vi "CAN_tester.vi"() -> ()   [LabVIEW 2017]
uses:
  <vilib>/nican/nican.llb/CanFrameTimed.ctl
panel:
  out "Frame to write":T1[](array[typedef]) {"Data" format="%.0x"; "ArbitrationId" format="%.0x"; "Timestamp" format="%<%I:%M:%S%3u %p\n%m/%d/%Y>T"}
  in  "Active":bool
  in  "Steering Control":T2={"Rot. sw 4"=1, "Rot. sw 5"=1, "Rot. sw 3"=1, "Rot. sw 1"=1, "Rot. sw 2"=1, "Button 3"=FALSE, "Button 1"=FALSE, "Button 2"=FALSE, "Button 4"=FALSE} {"Rot. sw 2" min=1 max=12 scale=1.0..12.0; "Rot. sw 1" min=1 max=12 scale=1.0..12.0; "Rot. sw 3" min=1 max=12 scale=1.0..12.0; "Rot. sw 5" min=1 max=12 scale=1.0..12.0; "Rot. sw 4" min=1 max=12 scale=1.0..12.0}
  in  "Brake Checked":T3 {"Brake Pressure Front" scale=0.0..100.0; "Brake Pressure Rear" scale=0.0..100.0}
  in  "Active":bool
  in  "AMK Setpoint FL":T4 {"AMK_Targetvelocity" scale=0.0..21500.0; "AMK_TorqueLimitPositive" scale=0.0..2140.0; "AMK_TorqueLimitNegative" scale=0.0..-2140.0}
  in  "Active":bool
  in  "AMK Setpoint RL":T4 {"AMK_Targetvelocity" scale=0.0..21500.0; "AMK_TorqueLimitPositive" scale=0.0..2140.0; "AMK_TorqueLimitNegative" scale=0.0..-2140.0}
  in  "Active":bool
  in  "AMK Setpoint FR":T4 {"AMK_Targetvelocity" scale=0.0..21500.0; "AMK_TorqueLimitPositive" scale=0.0..2140.0; "AMK_TorqueLimitNegative" scale=0.0..-2140.0}
  in  "Active":bool
  in  "AMK Setpoint FL":T4 {"AMK_Targetvelocity" scale=0.0..21500.0; "AMK_TorqueLimitPositive" scale=0.0..2140.0; "AMK_TorqueLimitNegative" scale=0.0..-2140.0}
  in  "Active":bool
  in  "Active":bool
  in  "ThrottleSteering":T5 {"APPS2" scale=0.0..100.0; "APPS1" scale=0.0..100.0; "Steering Angle 2" scale=90.0..-90.0; "Steering Angle 1" scale=90.0..-90.0}
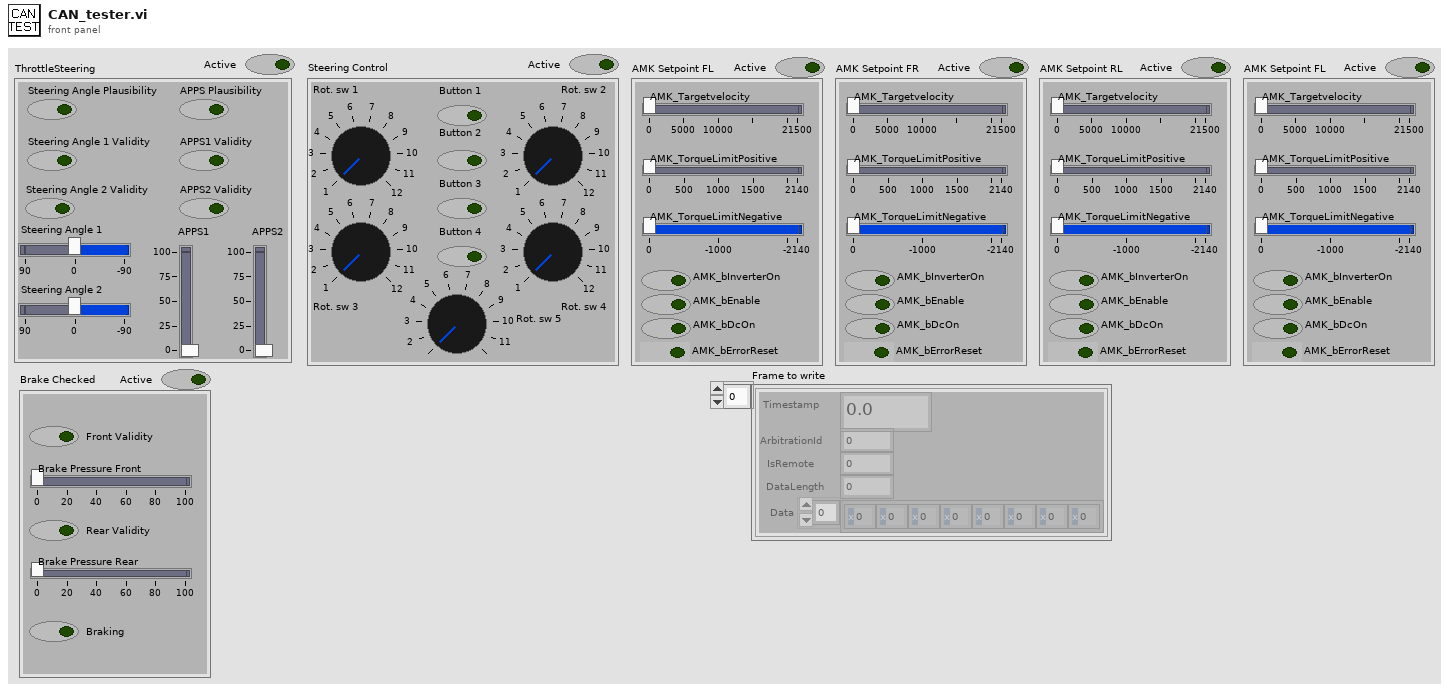
[diagram p1: front panel]
types:
  T1 = typedef "CanFrameTimed.ctl" = cluster{"Timestamp":dbl, "ArbitrationId":u32, "IsRemote":u8, "DataLength":u8, "Data":u8[]}
  T2 = cluster{"Rot. sw 4":u16, "Rot. sw 5":u16, "Rot. sw 3":u16, "Rot. sw 1":u16, "Rot. sw 2":u16, "Button 3":bool, "Button 1":bool, "Button 2":bool, "Button 4":bool}
  T3 = cluster{"Rear Validity":bool, "Front Validity":bool, "Brake Pressure Rear":dbl, "Brake Pressure Front":dbl, "Braking":bool}
  T4 = cluster{"AMK_bErrorReset":bool, "AMK_bDcOn":bool, "AMK_bEnable ":bool, "AMK_bInverterOn":bool, "AMK_TorqueLimitNegative":dbl, "AMK_TorqueLimitPositive":dbl, "AMK_Targetvelocity":dbl}
  T5 = cluster{"APPS Plausibility":bool, "Steering Angle 1":dbl, "Steering Angle 2":dbl, "APPS1":dbl, "APPS2":dbl, "APPS1 Validity":bool, "APPS2 Validity":bool, "Steering Angle Plausibility":bool, "Steering Angle 1 Validity":bool, "Steering Angle 2 Validity":bool}
  T6 = typedef "xobjhandle.ctl" = u32
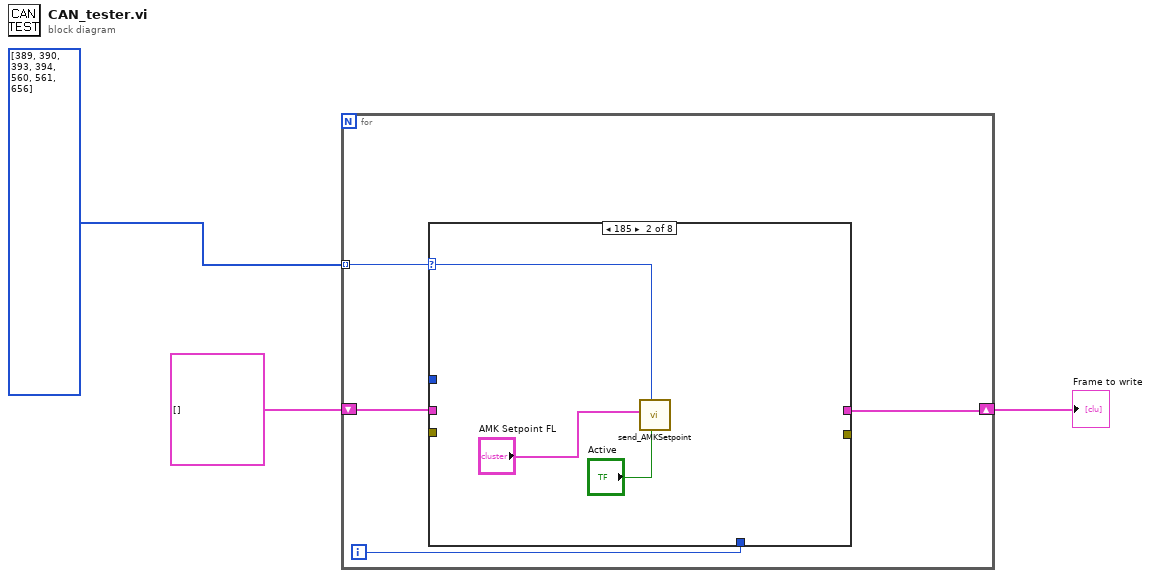
[diagram p0: block diagram]
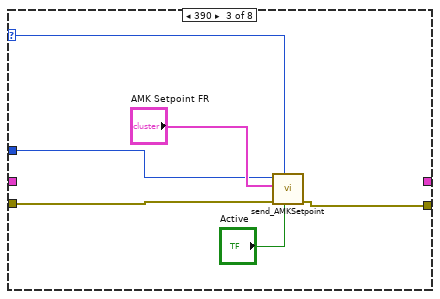
[diagram p3: hidden frame]
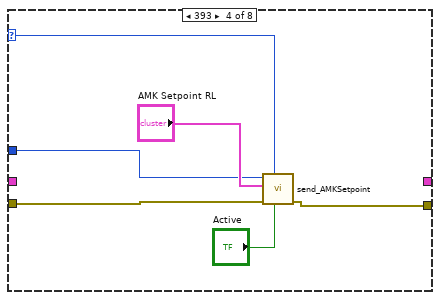
[diagram p4: hidden frame]
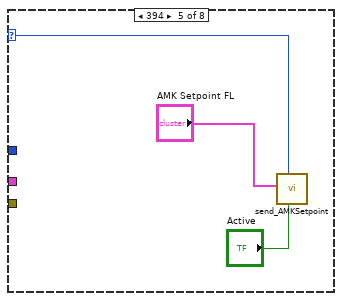
[diagram p5: hidden frame]
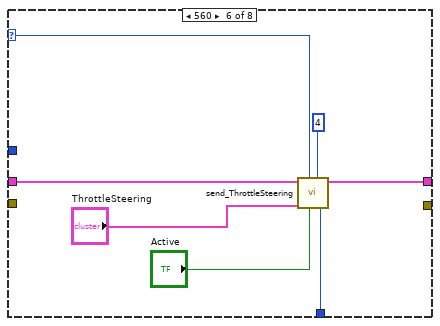
[diagram p6: hidden frame]
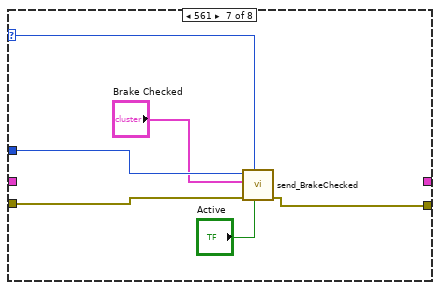
[diagram p7: hidden frame]
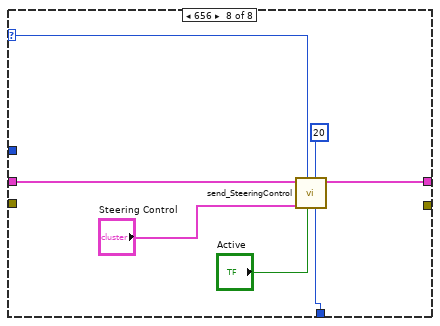
[diagram p8: hidden frame]
diagram:
  n1 = for {
    tunnel: u32[] [389, 390, 393, 394, 560, 561, 656] -> [w7] mode=indexing
    shift-right: [w5] -> w1
    shift-left: T1[] [] ("CAN frame") -> [w6]
    i -> [w4]
    n2 = case shown="185" w7 {
      selector: w7 -> [_ w9 w12 w19 w26 w34 w36 w49]
      tunnel: _ -> [_ _ w16 w22 _ _ w40 _]
      tunnel: [_ _ w13 w20 _ _ w41 _] -> _
      tunnel: _ -> [_ _ w15 w21 _ _ w39 _]
      tunnel: [w8 _ _ _ _ w33 _ w43] -> w5
      tunnel: w6 -> [w8 _ _ _ _ w31 _ w45]
      tunnel: w4 -> [_ _ _ _ _ w29 _ w47]
      frame 0, Default {
      }
      frame 389 {
        n3 = call "send_AMKSetpoint.vi"("Active"="Active", "ID"=w9, "Message"="AMK Setpoint FL") -> ()  [unwired: 7 in, 2 out]
      }
      frame 390 {
        n4 = call "send_AMKSetpoint.vi"("Active"="Active", "ID"=w12, "Error in"=w15, "Message"="AMK Setpoint FR", "ObjHandle in"=w16) -> ("Error out"=w13:errorcluster, "ObjHandle out"=w14:T6)  [unwired: 5 in]
      }
      frame 393 {
        n5 = call "send_AMKSetpoint.vi"("Active"="Active", "ID"=w19, "Error in"=w21, "Message"="AMK Setpoint RL", "ObjHandle in"=w22) -> ("Error out"=w20:errorcluster, "ObjHandle out"=w23:T6)  [unwired: 5 in]
      }
      frame 394 {
        n6 = call "send_AMKSetpoint.vi"("Active"="Active", "ID"=w26, "Message"="AMK Setpoint FL") -> ()  [unwired: 7 in, 2 out]
      }
      frame 560 {
        n7 = call "send_ThrottleSteering.vi"("Counter"=w29, "200/freq"=4, "Active"="Active", "CAN ID"=w34, "Message"="ThrottleSteering", "CAN frame"=w31) -> ("CAN frame out"=w33:T1[])  [unwired: 5 in]
      }
      frame 561 {
        n8 = call "send_BrakeChecked.vi"("Active"="Active", "ID"=w36, "Error in"=w39, "Message"="Brake Checked", "ObjHandle in"=w40) -> ("Error out"=w41:errorcluster, "ObjHandle out"=w42:T6)  [unwired: 5 in]
      }
      frame 656 {
        n9 = call "send_SteeringControl.vi"("Counter"=w47, "200/freq"=20, "Active 2"="Active", "CAN ID"=w49, "Message 2"="Steering Control", "CAN frame"=w45) -> ("CAN frame out"=w43:T1[])  [unwired: 5 in]
      }
    }
  }
  "Frame to write" <- w1
